vi "Example of Arrays to JSON.vi"() -> ()   [LabVIEW 2017]
uses:
  2bd85c31-efc5-4a81-bc2d-e57801eae9cd.vi
  Variant to JSON Text.vi
panel:
  out "Time per DBL":dbl[](array[numeric]) format="%#_3p"
  out "Time":dbl[](array[numeric]) format="%#_3p"
  out "<JSON>":string
  in  "Number in array":i32=10000
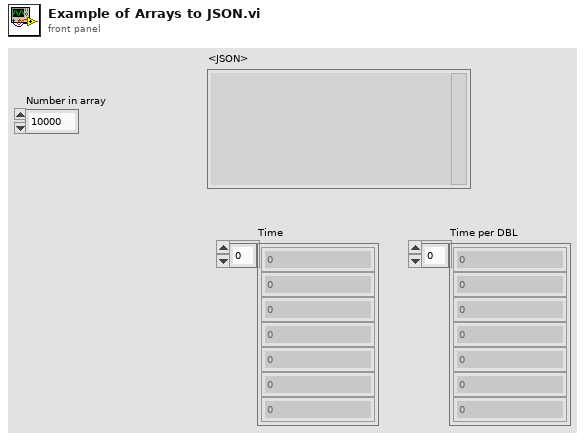
[diagram p1: front panel]
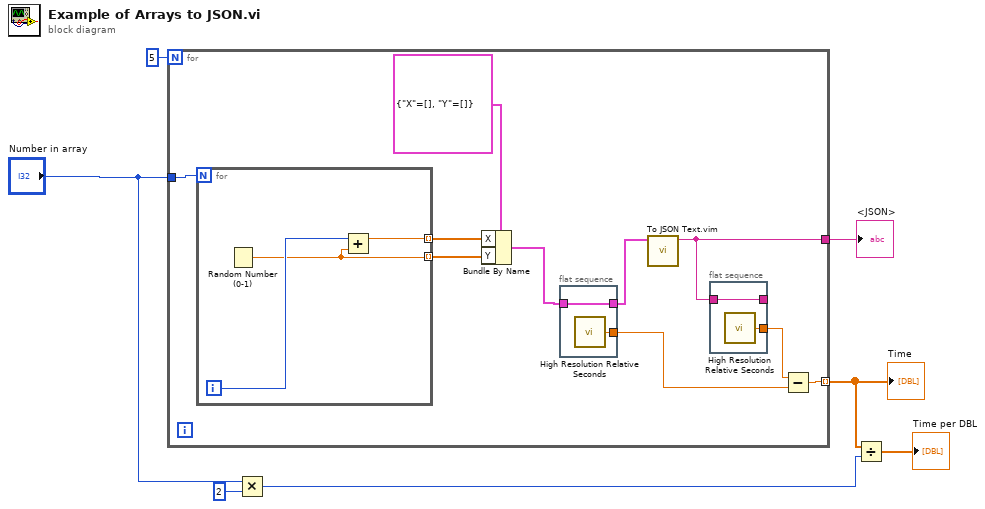
[diagram p0: block diagram]
diagram:
  n1 = for {
    N: 5 -> [_]
    tunnel: "Number in array" -> [w17]
    tunnel: [w11] -> w7
    tunnel: [w8] -> w5 mode=indexing
    n2 = for {
      N: w17 -> [_]
      tunnel: [w22] -> w15 mode=indexing
      tunnel: [w23] -> w16 mode=indexing
      i -> [w24]
      n3 = Random Number (0-1)() -> (number: 0 to 1=w22:dbl)
      n4 = Add(x=w24, y=w22) -> (x+y=w23:dbl)
    }
    n5 = Bundle By Name(cluster=cluster{"X":dbl[], "Y":dbl[]} {"X"=[], "Y"=[]}, "X"=w16, "Y"=w15) -> (w13:cluster{"X":dbl[], "Y":dbl[]})
    n6 = flat-sequence {
      tunnel: [w21] -> w12
      tunnel: w13 -> [w21]
      tunnel: [w20] -> w9
      frame #0 {
        n7 = call <vilib>:"High Resolution Relative Seconds.vi"() -> ("relative seconds"=w20:dbl)
      }
    }
    n8 = call "To JSON Text.vim"("Variant"=w12) -> ("<JSON>"=w11:string)  [unwired: 9 in, 1 out]
    n9 = flat-sequence {
      tunnel: [w19] -> _
      tunnel: w11 -> [w19]
      tunnel: [w18] -> w10
      frame #0 {
        n10 = call <vilib>:"High Resolution Relative Seconds.vi"() -> ("relative seconds"=w18:dbl)
      }
    }
    n11 = Subtract(x=w10, y=w9) -> (x-y=w8:dbl)
  }
  "<JSON>" <- w7
  "Time" <- w5
  n12 = Multiply(x="Number in array", y=2) -> (x*y=w2:i32)
  n13 = Divide(x=w5, y=w2) -> (x/y=→"Time per DBL":dbl[])
